vi "Get Device Information.vi"() -> ()   [LabVIEW 2018]
uses:
  TwinCAT ADS Class/Controls/Device Information.ctl
  TwinCAT ADS Class/TwinCAT ADS.lvclass
panel:
  out "Device Infomation":T1
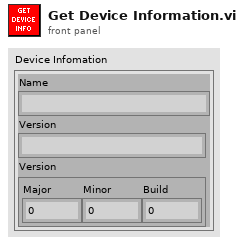
[diagram p1: front panel]
types:
  T1 = typedef "TwinCAT ADS.lvclass/Device Information.ctl" = cluster{"Name":string, "Version":string, "Version":cluster{"Major":i32, "Minor":i32, "Build":i32}}
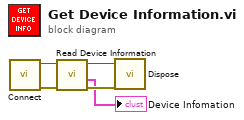
[diagram p0: block diagram]
diagram:
  n1 = call "Connect.vi"() -> ("error out"=w5:errorcluster, "TwinCAT ADS out"=w4:refnum<class "TwinCAT ADS.lvclass">)  [unwired: 10 in]
  n2 = call "Read Device Information.vi"("error in (no error)"=w5, "TwinCAT ADS in"=w4) -> ("error out"=w2:errorcluster, "Device Information"=→"Device Infomation":T1, "TwinCAT ADS out"=w3:refnum<class "TwinCAT ADS.lvclass">)  [unwired: 7 in]
  n3 = call "Dispose.vi"("error in (no error)"=w2, "TwinCAT ADS in"=w3) -> ()  [unwired: 9 in, 1 out]
